vi "(SUBTASK 4) - Drop off.vi"() -> ()   [LabVIEW 2016, in "testrobot.lvrbt"]
uses:
  testrobot.lvrbt
  <vilib>/NXT/Subs/LVHSConnector.ctl
  <vilib>/NXT/LegoClasses/BrickReference/BrickReference.lvclass
  <vilib>/NXT/Block Support/NXT_InputPort.ctl
  <vilib>/NXT/Block Support/NXT_OutputPort.ctl
panel:
  out "Scaled dif 2":dbl
  in  "Port (Port 1)":T1=1 items=["Port 1", "Port 2", "Port 3", "Port 4"]
  out "Distance":dbl
  in  "ultra":T1=2 items=["Port 1", "Port 2", "Port 3", "Port 4"]
  in  "left light":T1 items=["Port 1", "Port 2", "Port 3", "Port 4"]
  in  "right light":T1=3 items=["Port 1", "Port 2", "Port 3", "Port 4"]
  out "only right":bool
  out "both negative":bool
  out "both positve":bool
  out "Left":bool
  out "Right":bool
  out "forward":bool
  out "Right 2":sgl
  out "Left 2":sgl
  out "NXT/EV3 2":T2
  in  "NXT/EV3":T2
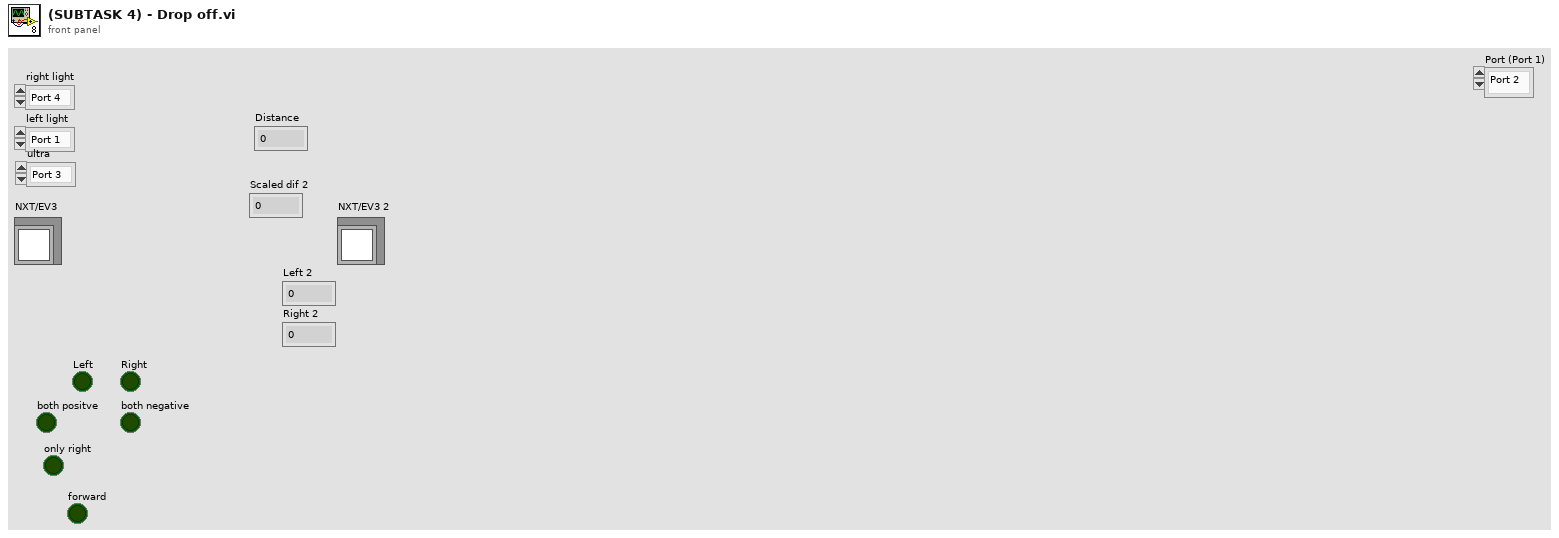
[diagram p1: front panel]
types:
  T1 = typedef "NXT_InputPort.ctl" = u32
  T2 = typedef "LVHSConnector.ctl" = refnum<class "BrickReference.lvclass">
  T3 = typedef "NXT_OutputPort.ctl" = u8
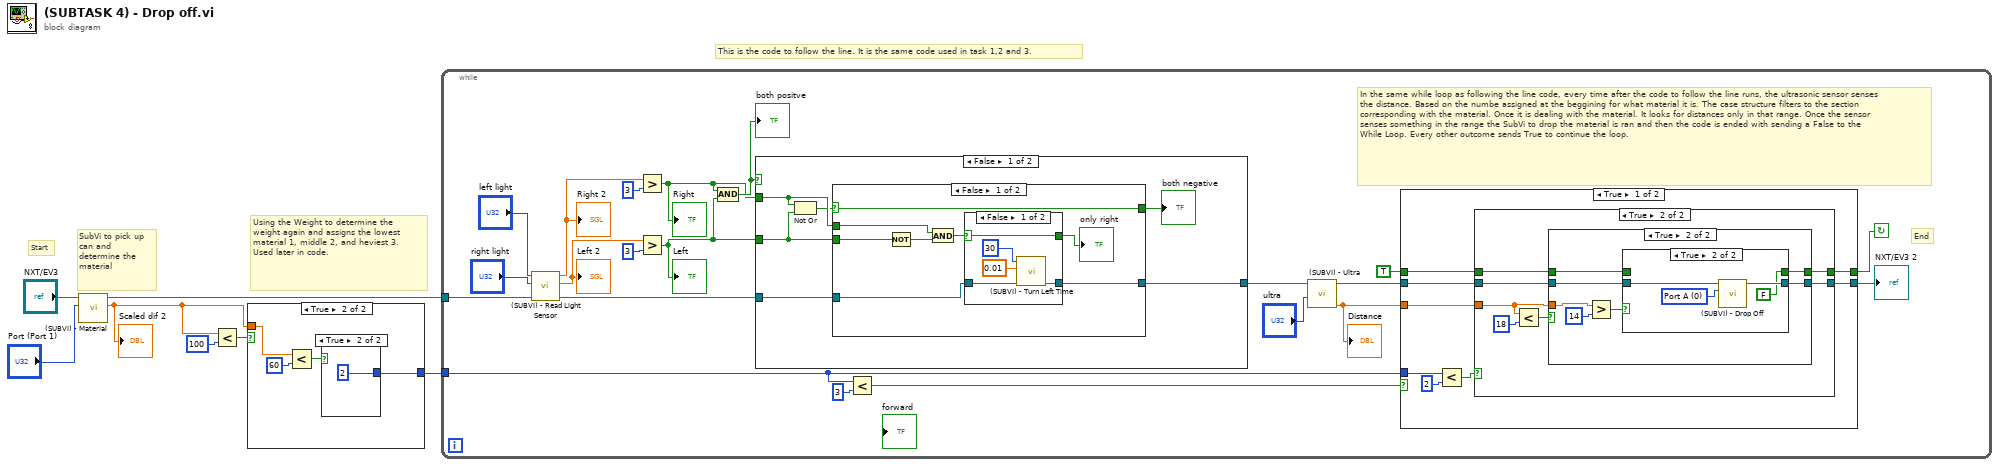
[diagram p0: block diagram]
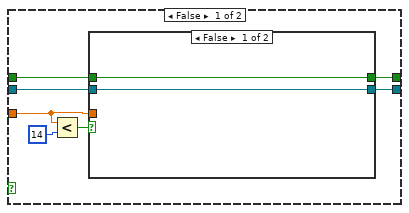
[diagram p2: hidden frame]
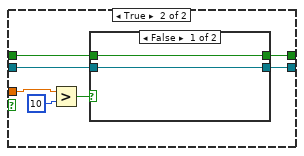
[diagram p3: hidden frame]
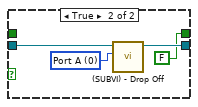
[diagram p4: hidden frame]
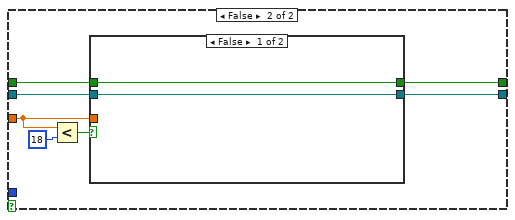
[diagram p7: hidden frame]
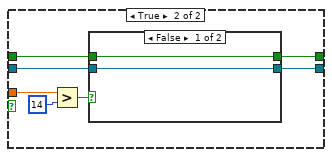
[diagram p8: hidden frame]
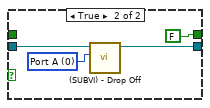
[diagram p9: hidden frame]
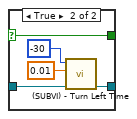
[diagram p10: hidden frame]
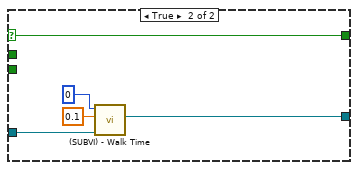
[diagram p11: hidden frame]
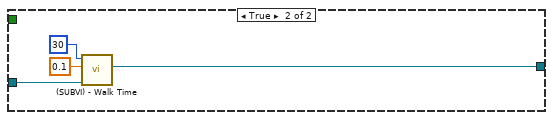
[diagram p12: hidden frame]
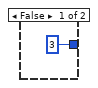
[diagram p13: hidden frame]
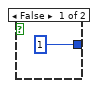
[diagram p14: hidden frame]
diagram:
  # "This is the code to follow the line. It is the same code used in task 1,2 and 3."
  # "Using the Weight to determine the weight again and assigns the lowest material 1, middle 2, and heviest 3. Used later in code."
  # "SubVi to pick up can and determine the material"
  # "Start"
  n1 = call "(SUBVI) - Material.vi"("Port (Port 1)"="Port (Port 1)", "NXT/EV3"="NXT/EV3") -> ("Scaled dif"=w3:dbl, "NXT/EV3 2"=w2:T2)  [unwired: 8 in]
  "Scaled dif 2" <- w3
  n2 = Less?(x=w3, y=100) -> (x < y?=w4:bool)
  n3 = case shown="True" w4 {
    tunnel: w3 -> [_ w12]
    tunnel: [3 w9] -> w1
    frame False {
    }
    frame True {
      n4 = Less?(x=w12, y=60) -> (x < y?=w11:bool)
      n5 = case shown="True" w11 {
        tunnel: [1 2] -> w9
        frame False {
        }
        frame True {
        }
      }
    }
  }
  n6 = while {
    tunnel: w2 -> [w24]
    tunnel: w1 -> [w20]
    stop <- w16 continue-if-true
    # "End"
    # "In the same while loop as following the line code, every time after the code to follow the line runs, the ultrasonic sensor senses the distance. Based on the numbe assigned at the beggining for what material it is. The case structure filters to the section corresponding with the material. Once it is dealing with the material. It looks for distances only in that range. Once the sensor senses something in the range the SubVi to drop the material is ran and then the code is ended with sending a False to the While Loop. Every other outcome sends True to continue the loop."
    n7 = call "(SUBVI) - Read Light Sensor.vi"("NXT/EV3"=w24, "Port (Port 1) 2"="right light", "Port (Port 1)"="left light") -> ("NXT/EV3 2"=w30:T2, "Scaled Value 2"=w33:sgl, "Scaled Value"=w32:sgl)  [unwired: 6 in]
    "Left 2" <- w33
    "Right 2" <- w32
    n8 = Greater?(x=w32, y=3) -> (0:w29:bool)
    "Right" <- w29
    n9 = Greater?(x=w33, y=3) -> (0:w28:bool)
    "Left" <- w28
    n10 = And(x=w29, y=w28) -> (x .and. y?=w31:bool)
    "both positve" <- w31
    n11 = case shown="False" w31 {
      tunnel: w30 -> [w111 w140]
      tunnel: [w110 w139] -> w25
      tunnel: w29 -> [w114 _]
      tunnel: w28 -> [w113 _]
      frame False {
        n12 = Not Or(1:w113, 2:w114) -> (0:w112:bool)
        n13 = case shown="False" w112 {
          selector: w112 -> [w123 w138]
          tunnel: [w123 w138] -> w115
          tunnel: w114 -> [w121 _]
          tunnel: w113 -> [w119 _]
          tunnel: w111 -> [w117 w135]
          tunnel: [w116 w134] -> w110
          frame False {
            n14 = Not(x=w119) -> (.not. x?=w120:bool)
            n15 = And(x=w121, y=w120) -> (x .and. y?=w122:bool)
            n16 = case shown="False" w122 {
              selector: w122 -> [w128 w133]
              tunnel: [w128 w133] -> w118
              tunnel: w117 -> [w125 w130]
              tunnel: [w124 w129] -> w116
              frame False {
                n17 = call "(SUBVI) - Turn Left Time.vi"("NXT/EV3"=w125, "Time walking"=0.01, "Walk Speed"=30) -> ("NXT/EV3 2"=w124:T2)  [unwired: 8 in]
              }
              frame True {
                n18 = call "(SUBVI) - Turn Left Time.vi"("NXT/EV3"=w130, "Time walking"=0.01, "Walk Speed"=-30) -> ("NXT/EV3 2"=w129:T2)  [unwired: 8 in]
              }
            }
            "only right" <- w118
          }
          frame True {
            n19 = call "(SUBVI) - Walk Time.vi"("NXT/EV3"=w135, "Time walking"=0.1, "Walk Speed"=0) -> ("NXT/EV3 2"=w134:T2)  [unwired: 8 in]
          }
        }
        "both negative" <- w115
      }
      frame True {
        n20 = call "(SUBVI) - Walk Time.vi"("NXT/EV3"=w140, "Time walking"=0.1, "Walk Speed"=30) -> ("NXT/EV3 2"=w139:T2)  [unwired: 8 in]
      }
    }
    n21 = Less?(x=w20, y=3) -> (x < y?=w21:bool)
    n22 = call "(SUBVI) - Ultra.vi"("Port (Port 1)"="ultra", "NXT/EV3"=w25) -> ("Inches"=w18:sgl, "NXT/EV3 2"=w23:T2)  [unwired: 8 in]
    "Distance" <- w18
    n23 = case shown="True" w21 {
      tunnel: w23 -> [w39 w91]
      tunnel: w20 -> [w43 _]
      tunnel: w18 -> [w40 w92]
      tunnel: [w38 w90] -> w17
      tunnel: [w37 w89] -> w16
      tunnel: TRUE -> [w36 w88]
      frame True {
        n24 = Less?(x=w43, y=2) -> (x < y?=w41:bool)
        n25 = case shown="True" w41 {
          tunnel: w40 -> [w47 w70]
          tunnel: w39 -> [w48 w69]
          tunnel: [w46 w68] -> w38
          tunnel: [w45 w67] -> w37
          tunnel: w36 -> [w44 w66]
          frame False {
            n26 = Less?(x=w47, y=14) -> (x < y?=w50:bool)
            n27 = case shown="False" w50 {
              tunnel: w47 -> [_ w58]
              tunnel: w48 -> [w52 w56]
              tunnel: [w52 w55] -> w46
              tunnel: [w51 w54] -> w45
              tunnel: w44 -> [w51 w53]
              frame False {
              }
              frame True {
                n28 = Greater?(x=w58, y=10) -> (0:w57:bool)
                n29 = case shown="False" w57 {
                  tunnel: w56 -> [w61 w65]
                  tunnel: [w61 w64] -> w55
                  tunnel: [w60 FALSE] -> w54
                  tunnel: w53 -> [w60 _]
                  frame False {
                  }
                  frame True {
                    w63 = T3 0 items=["Port A", "Port B", "Port C", "Port D"] ("Motors")
                    n30 = call "(SUBVI) - Drop Off.vi"("Motors"=w63, "NXT/EV3"=w65) -> ("NXT/EV3 2"=w64:T2)  [unwired: 9 in]
                  }
                }
              }
            }
          }
          frame True {
            n31 = Less?(x=w70, y=18) -> (x < y?=w71:bool)
            n32 = case shown="True" w71 {
              tunnel: w70 -> [_ w80]
              tunnel: w69 -> [w74 w78]
              tunnel: [w74 w77] -> w68
              tunnel: [w73 w76] -> w67
              tunnel: w66 -> [w73 w75]
              frame False {
              }
              frame True {
                n33 = Greater?(x=w80, y=14) -> (0:w79:bool)
                n34 = case shown="True" w79 {
                  tunnel: w78 -> [w83 w87]
                  tunnel: [w83 w86] -> w77
                  tunnel: [w82 FALSE] -> w76
                  tunnel: w75 -> [w82 _]
                  frame False {
                  }
                  frame True {
                    w85 = T3 0 items=["Port A", "Port B", "Port C", "Port D"] ("Motors")
                    n35 = call "(SUBVI) - Drop Off.vi"("Motors"=w85, "NXT/EV3"=w87) -> ("NXT/EV3 2"=w86:T2)  [unwired: 9 in]
                  }
                }
              }
            }
          }
        }
      }
      frame False {
        n36 = Less?(x=w92, y=18) -> (x < y?=w93:bool)
        n37 = case shown="False" w93 {
          tunnel: w92 -> [_ w103]
          tunnel: w91 -> [w96 w100]
          tunnel: [w96 w99] -> w90
          tunnel: [w95 w98] -> w89
          tunnel: w88 -> [w95 w97]
          frame False {
          }
          frame True {
            n38 = Greater?(x=w103, y=14) -> (0:w101:bool)
            n39 = case shown="False" w101 {
              tunnel: w100 -> [w105 w109]
              tunnel: [w105 w108] -> w99
              tunnel: [w104 FALSE] -> w98
              tunnel: w97 -> [w104 _]
              frame False {
              }
              frame True {
                w107 = T3 0 items=["Port A", "Port B", "Port C", "Port D"] ("Motors")
                n40 = call "(SUBVI) - Drop Off.vi"("Motors"=w107, "NXT/EV3"=w109) -> ("NXT/EV3 2"=w108:T2)  [unwired: 9 in]
              }
            }
          }
        }
      }
    }
    "NXT/EV3 2" <- w17
  }
